vi "Main.vi"() -> ()   [LabVIEW 2020]
doc: "This template is for the Queued Message Handler design pattern.\n\nThe Event Handling Loop generates messages based on user interface actions.\n\nThe Message Handling Loop processes messages generated by the Event Handling Loop, or by other messages. The messages are string values, so new messages can be added easily to the Message Cases case structure in the Message Handling Loop. Each message cluster can also provide an optional value for Message Data, which is a variant that can be converted to whatever message-specific data is required."
uses:
  controls/UI Data.ctl
  controls/Lock-in config.ctl
  controls/Mono config.ctl
  <vilib>/event_ctls.llb/lveventtype.ctl
  Lock-in-amplifier/Libraries/Lock-in amplifier/Support/Filter config -- cluster.ctl
  Lock-in-amplifier/Libraries/Lock-in amplifier/Support/Input signal config -- typedef.ctl
  Lock-in-amplifier/Libraries/Lock-in amplifier/Support/Sense-Reserve config -- cluster.ctl
  controls/Wake HL data -- cluster.ctl
  <vilib>/Utility/sysdir.llb/System Directory Type.ctl
  support/Message Queue/Enqueue Message (Single).vi
  <vilib>/Utility/error.llb/Error Cluster From Error Code.vi
  <vilib>/ErrorRing/Error Ring.xnode
  support/Message Queue/Message Queue.lvlib
  support/User Event - Stop/User Event - Stop.lvlib
  Lock-in-amplifier/Libraries/Lock-in amplifier/Lock-in amplifier.lvlib
  Monochromator/Libraries/Monochromator/Monochromator.lvlib
panel:
  in  "Export":bool
  out "Current measurement":dbl caption="Medición" format="%0.6fmV"
  in  "Continous acquisition":bool
  in  "Simulate \nmono?":bool
  out "Last measurement":dbl caption="Medición" format="%#_gmV"
  in  "Position":dbl caption="Posición" format="%#_gnm"
  in  "Move":bool
  in  "Interval":dbl=10.0 caption="Intervalo" format="%#_gnm"
  out "Current position":dbl caption="Posición actual" format="%#_gnm"
  in  "Stop acquisition":bool
  out "XY Graph":cluster{"X":dbl, "Y":dbl}[](graph)
  in  "N samples":i32=1 caption="Muestras"
  in  "Average":bool
  in  "Final wavelength":dbl=800.0 caption="Fin" format="%#_gnm"
  in  "Initial wavelength":dbl=400.0 caption="Inicio" format="%#_gnm"
  in  "Speed":dbl=100.0 caption="Velocidad" format="%#_gnm/min"
  in  "Start acquiring":bool
  in  "Simulate \nlock-in?":bool
  out "Mono connected":bool
  out "Lock-in connected":bool
  in  "Settings":bool
  out "Status":string caption="Estado"
  in  "Exit":bool
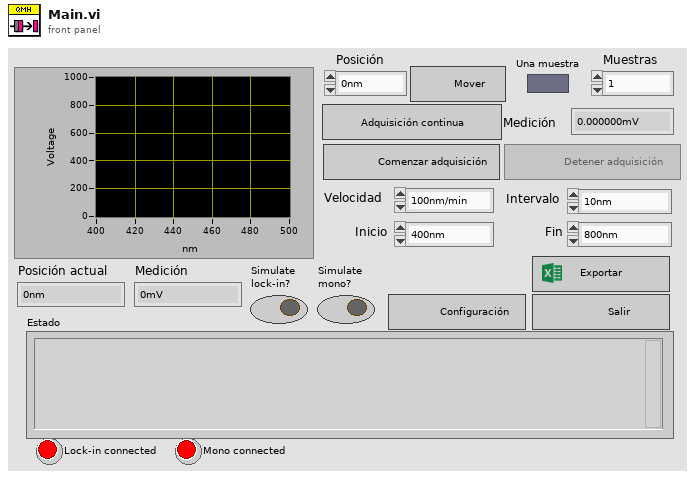
[diagram p1: front panel]
types:
  T1 = typedef "UI Data.ctl" = cluster{"Status":string, "Lockin Mod ID":i32, "Mono Mod ID":i32, "Lock-in config":T2, "Mono config":T3, "Lock-in connected?":bool, "Mono connected?":bool, "Data":cluster{"Position":dbl, "Value":dbl}[], "Manual move?":bool, "Current position":dbl, "Interval":dbl, "Operative?":bool}
  T2 = typedef "Lock-in config.ctl" = cluster{"VISA resource ":refnum<visa-resource-name>}
  T3 = typedef "Mono config.ctl" = cluster{"VISA resource ":refnum<visa-resource-name>, "nm/min":dbl}
  T4 = typedef "Lock-in amplifier.lvlib/Broadcast Events--cluster.ctl" = cluster{"Module Did Init":refnum<user-event>, "Status Updated":refnum<user-event>, "Error Reported":refnum<user-event>, "Module Did Stop":refnum<user-event>, "Update Module Execution Status":refnum<user-event>, "Helper Loop Status Updated":refnum<user-event>, "Data available":refnum<user-event>}
  T5 = typedef "Monochromator.lvlib/Broadcast Events--cluster.ctl" = cluster{"Module Did Init":refnum<user-event>, "Status Updated":refnum<user-event>, "Error Reported":refnum<user-event>, "Module Did Stop":refnum<user-event>, "Update Module Execution Status":refnum<user-event>, "Helper Loop Status Updated":refnum<user-event>, "Data read":refnum<user-event>, "GOTO ended":refnum<user-event>}
  T6 = cluster{"Stop Event":refnum<user-event>, "Wake HL":refnum<user-event>, "Stop HL":refnum<user-event>}
  T7 = typedef "Message Queue.lvlib/All Message Queues.ctl" = cluster{"UI":refnum<queue>}
  T8 = enum8{"Enabled", "Disabled", "Disabled and Grayed Out"}
  T9 = typedef "Wake HL data -- cluster.ctl" = cluster{"Mono Mod ID":i32, "Timeout":i32, "Wavelength":dbl}
  T10 = typedef "Lock-in amplifier.lvlib/Sense-Reserve config -- cluster.ctl" = cluster{"Dynamic Reserve ":i16, "Sensitivity":i16}
  T11 = typedef "Lock-in amplifier.lvlib/Input signal config -- typedef.ctl" = cluster{"Input Shield Grounding":u16, "Input Connection":u16, "Input Coupling":u16}
  T12 = typedef "Lock-in amplifier.lvlib/Filter config -- cluster.ctl" = cluster{"Time Constant":u16, "Enable Sync Filter?":bool, "Low Pass Filter Slope":u16}
  T13 = cluster{"baud rate":u32, "data bits":u16, "parity":enum16{"None", "Odd", "Even", "Mark", "Space"}, "stop bits":u16}
  T14 = typedef "System Directory Type.ctl" = i32
  T15 = typedef "lveventtype.ctl" = enum32{"Null", "Timeout", "Annotation Menu Selection", "Annotation Menu Selection?", "App Instance Close", "App Instance Close?", "Autoscale Range Change", "Bookmark Info Change", "Cell Edit", "Cell Edit?", "Cursor Grab", "Cursor Grab?", "Cursor Menu Selection", "Cursor Menu Selection?", "Cursor Move", "Cursor Release", "Data Change", "Direction Change", "Display State Change", "Drag Ended", "Drag Enter", "Drag Leave", "Drag Over", "Drag Source Update", "Drag Starting", "Drag Starting?", "Drop", "Exec State Change", "Key Down", "Key Down?", "Key Repeat", "Key Repeat?", "Key Up", "Listbox Double Click", "Menu Activation?", "Menu Selection (App)", "Menu Selection? (App)", "Menu Selection (User)", "Mouse Down", "Mouse Down?", "Mouse Enter", "Mouse Leave", "Mouse Move", "Mouse Up", "Mouse Wheel", "NI Security User Change (App)", "Pane Size", "Panel Close", "Panel Close?", "Panel Resize", "Plot Attribute Change", "Scale Range Change", "Shortcut Menu Activation?", "Shortcut Menu Selection (App)", "Shortcut Menu Selection? (App)", "Shortcut Menu Selection (User)", "Tree Double Click", "Tree Drag", "Tree Drag?", "Tree Drop", "Tree Drop?", "Tree Item Close", "Tree Item Close?", "Tree Item Open", "Tree Item Open?", "User Event", "Value Change"}
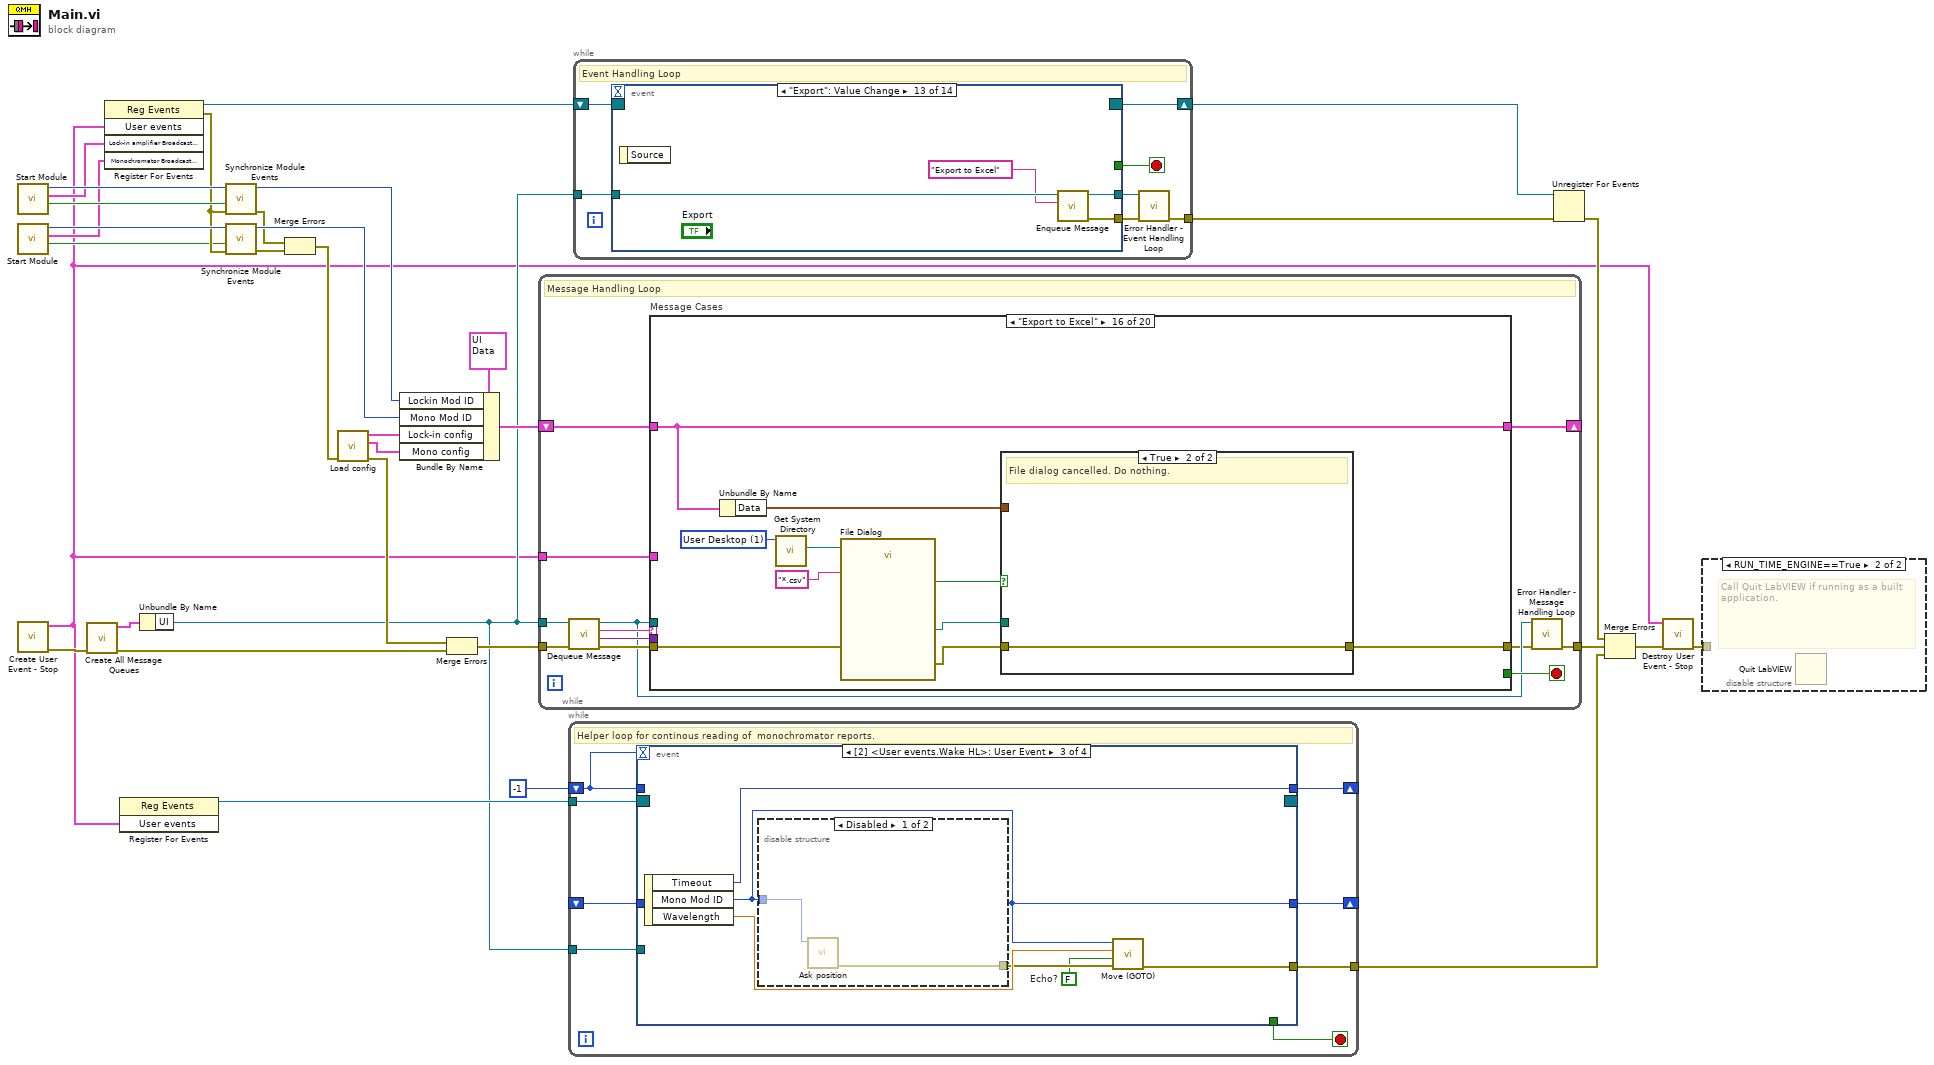
[diagram p0: block diagram]
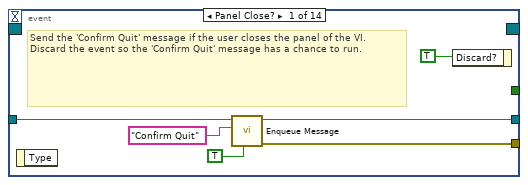
[diagram p2: hidden frame]
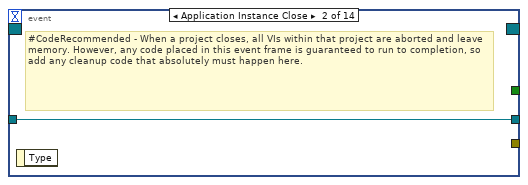
[diagram p3: hidden frame]
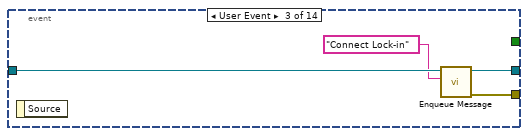
[diagram p4: hidden frame]
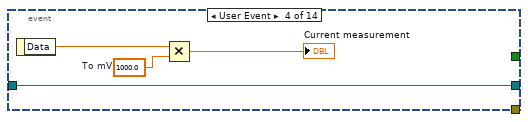
[diagram p5: hidden frame]
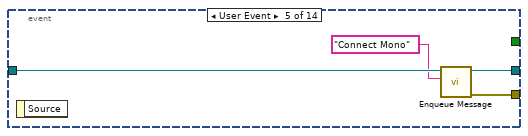
[diagram p6: hidden frame]
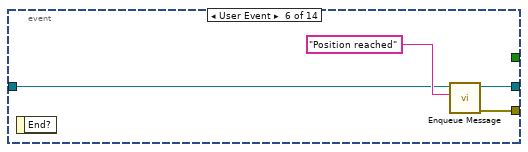
[diagram p7: hidden frame]
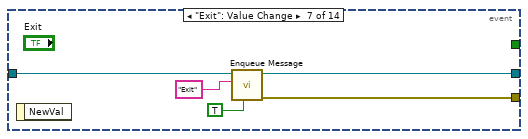
[diagram p8: hidden frame]
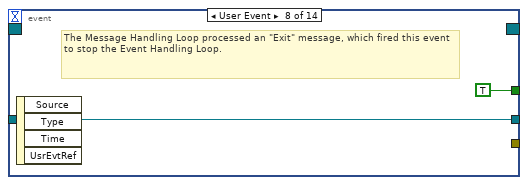
[diagram p9: hidden frame]
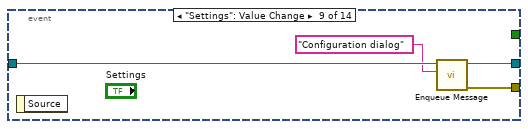
[diagram p10: hidden frame]
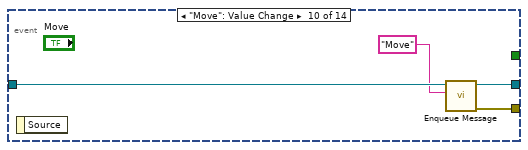
[diagram p11: hidden frame]
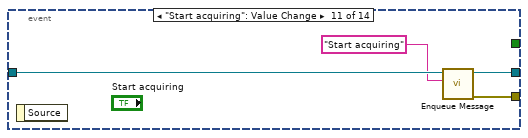
[diagram p12: hidden frame]
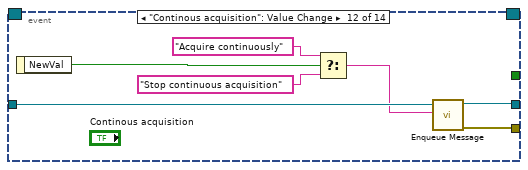
[diagram p13: hidden frame]
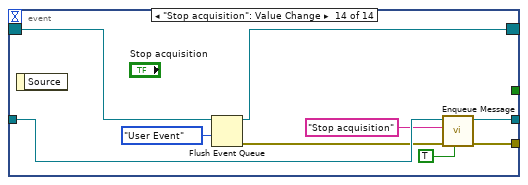
[diagram p14: hidden frame]
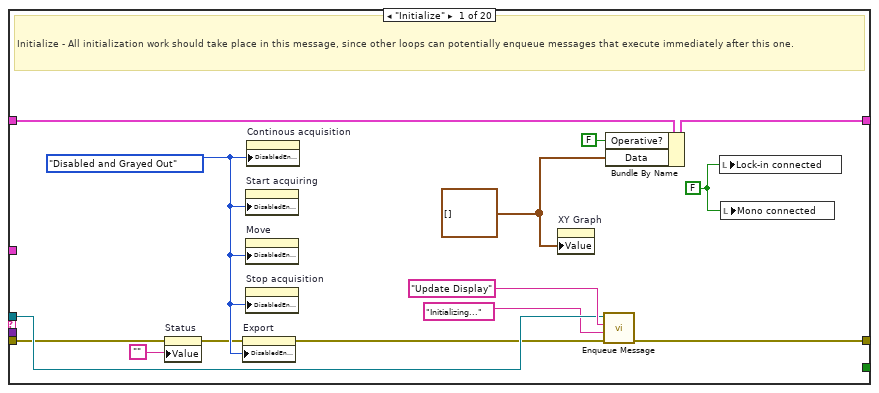
[diagram p15: hidden frame]
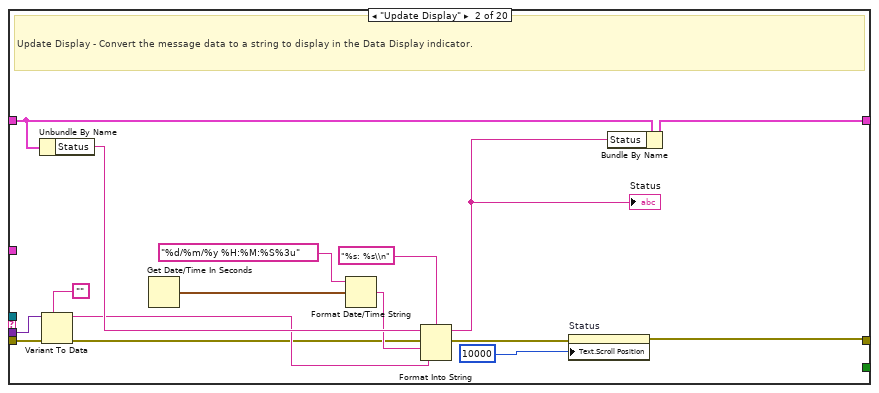
[diagram p16: hidden frame]
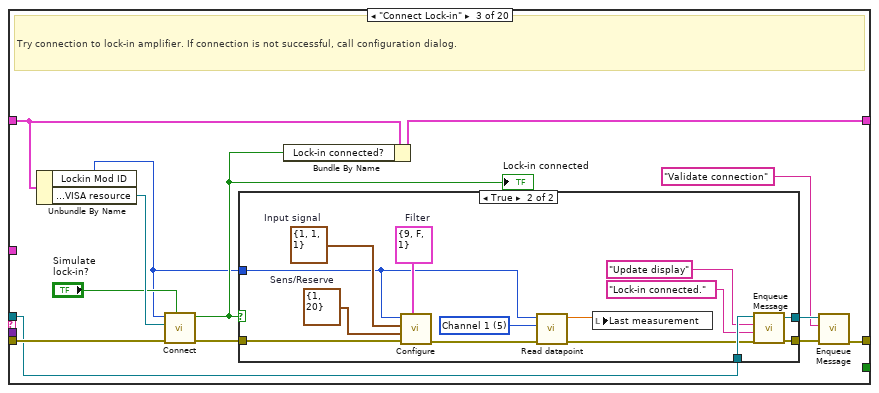
[diagram p17: hidden frame]
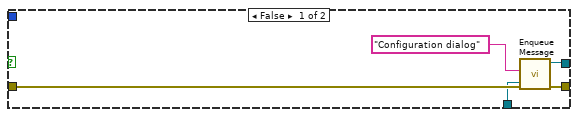
[diagram p18: hidden frame]
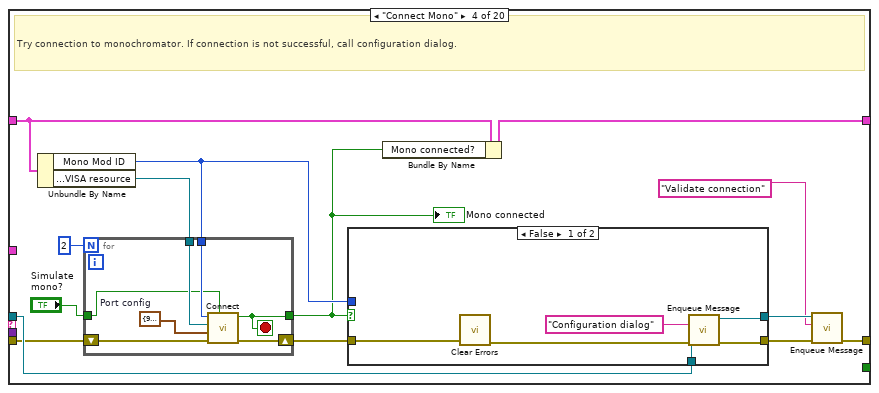
[diagram p19: hidden frame]
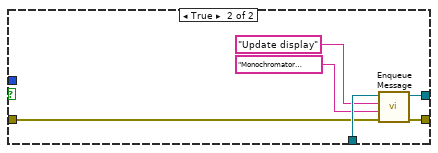
[diagram p20: hidden frame]
diagram:
  n1 = call "Start Module.vi"() -> ("Wait for Event Sync?"=w21:bool, "Lock-in amplifier Broadcast Events"=w20:T4, "Module ID"=w22:i32)  [unwired: 8 in, 1 out]
  n2 = call "Start Module.vi"() -> ("Wait for Event Sync?"=w16:bool, "Monochromator Broadcast Events"=w17:T5, "Module ID"=w19:i32)  [unwired: 8 in, 1 out]
  n3 = call "Create User Event - Stop.vi"() -> ("error out"=w30:errorcluster, "User events"=w1:T6)  [unwired: 10 in]
  n4 = call "Create All Message Queues.vi"("error in (no error)"=w30) -> ("error out"=w33:errorcluster, "Message Queues out"=w32:T7)  [unwired: 9 in]
  n5 = register-events(w1, w20, w17) -> (reference out=w24:refnum<event-registration>, error out=w18:errorcluster)  [unwired: 2 in]
  n6 = register-events(w1) -> (reference out=w4:refnum<event-registration>)  [unwired: 2 in, 1 out]
  n7 = Unbundle By Name(w32) -> ("UI"=w3:refnum<queue>)
  n8 = call "Synchronize Module Events.vi"("error in"=w18, "Wait for Event Sync?"=w21, "Module ID in"=w22) -> ("error out"=w11:errorcluster, "Module ID out"=w13:i32)  [unwired: 7 in]
  n9 = call "Synchronize Module Events.vi"("error in"=w18, "Wait for Event Sync?"=w16, "Module ID in"=w19) -> ("error out"=w10:errorcluster, "Module ID out"=w12:i32)  [unwired: 7 in]
  n10 = Merge Errors(w11, w10) -> (w9:errorcluster)
  n11 = call "Load config.vi"("error in (no error)"=w9) -> ("error out"=w8:errorcluster, "Mono config"=w6:T3, "Lock-in config"=w7:T2)  [unwired: 8 in]
  n12 = Bundle By Name(cluster=T1 {"Status"="", "Lockin Mod ID"=-1, "Mono Mod ID"=-1, "Lock-in config"={"VISA resource "=""}, "Mono config"={"VISA resource "="", "nm/min"=0.0}, "Lock-in connected?"=FALSE, "Mono connected?"=FALSE, "Data"=[], "Manual move?"=FALSE, "Current position"=0.0, "Interval"=0.0, "Operative?"=FALSE} ("Data Cluster"), "Lockin Mod ID"=w13, "Mono Mod ID"=w12, "Lock-in config"=w7, "Mono config"=w6) -> (w14:T1)
  n13 = Merge Errors(w8, w33) -> (w23:errorcluster)
  n14 = while {
    tunnel: w3 -> [w37]
    shift-right: [w44] -> _
    shift-left: w14 -> [w45]
    tunnel: w1 -> [w42]
    tunnel: w23 -> [w41]
    tunnel: [w35] -> w31
    stop <- w43 stop-if-true
    # "Message Handling Loop"
    n15 = call "Dequeue Message.vi"("error in (no error)"=w41, "Message Queue"=w37) -> ("error out"=w40:errorcluster, "Message Data"=w38:variant, "Message"=w39:string, "dup Message Queue"=w36:refnum<queue>)  [unwired: 6 in]
    n16 = case "Message Cases" shown="\"Export to Excel\"" w39 {
      selector: w39 -> [_ _ _ _ _ _ _ _ _ _ _ _ _ _ _ _ _ _ _ w392]
      tunnel: w36 -> [w57 _ w85 w121 w147 w175 w209 w233 _ _ _ w270 w285 w296 w323 _ _ w372 w391 _]
      tunnel: w40 -> [w51 w75 w88 w120 w149 w180 w222 w230 w248 w253 w257 w267 w294 w305 w333 w357 w369 w376 w387 _]
      tunnel: [w59 w65 w78 w111 w148 w174 w210 w234 w247 w252 w262 w271 w291 w304 w332 w351 w363 w374 w388 w393] -> w34
      tunnel: w45 -> [w55 w63 w84 w116 w143 w182 w214 w229 w246 w251 w260 w264 w282 w300 w336 w350 w368 w375 w380 w394]
      tunnel: [w53 w62 w83 w115 w142 w181 w212 w229 w246 w251 w258 w263 w282 w302 w334 w350 w368 w375 w380 w394] -> w44
      tunnel: [_ _ _ _ _ _ _ _ _ _ _ _ _ _ _ _ _ _ TRUE _] -> w43
      tunnel: w38 -> [_ w74 _ _ _ _ _ _ _ _ _ _ _ _ w329 _ w367 _ w384 _]
      tunnel: w42 -> [_ _ _ _ _ _ w220 _ _ _ _ _ w295 w301 w330 _ _ _ w377 _]
      frame "Initialize" {
        w52 = FALSE ("Lock-in connected")
        w48 = T8."Disabled and Grayed Out" ("Disabled")
        w54 = cluster{"Position":dbl, "Value":dbl}[] [] ("Data")
        # "Initialize - All initialization work should take place in this message, since other loops can potentially enqueue messages that execute immediately after this one."
        n17 = property on="Status" class="Str"(error in=w51, "Value"="") -> (error out=w47:errorcluster)  [unwired: 1 in, 1 out]
        n18 = property on="Export" class="Bool"(error in=w47, "DisabledEnum"=w48) -> (error out=w46:errorcluster)  [unwired: 1 in, 1 out]
        n19 = property on="Start acquiring" class="Bool"("DisabledEnum"=w48) -> ()  [unwired: 2 in, 2 out]
        n20 = property on="Move" class="Bool"("DisabledEnum"=w48) -> ()  [unwired: 2 in, 2 out]
        n21 = property on="Stop acquisition" class="Bool"("DisabledEnum"=w48) -> ()  [unwired: 2 in, 2 out]
        n22 = property on="Continous acquisition" class="Bool (strict)"("DisabledEnum"=w48) -> ()  [unwired: 2 in, 2 out]
        n23 = property on="XY Graph" class="XYGraph (strict)"("Value"=w54) -> ()  [unwired: 2 in, 2 out]
        n24 = call-poly "Enqueue Message.vi"("error in (no error)"=w46, "Message Data"="Initializing..." ("Initial Message"), "Message"="Update Display", "Message Queue"=w57) -> ("error out"=w59:errorcluster)  [unwired: 6 in, 1 out]
        n25 = Bundle By Name(cluster=w55, "Operative?"=FALSE, "Data"=w54) -> (w53:T1)
        n26 = local write "Lock-in connected"(w52) -> ()
        n27 = local write "Mono connected"(w52) -> ()
      }
      frame "Update Display" {
        # "Update Display - Convert the message data to a string to display in the Data Display indicator."
        n28 = Unbundle By Name(w63) -> ("Status"=w72:string)
        n29 = Variant To Data(error in=w75, type="", Variant=w74) -> (data=w68:string, error out=w67:errorcluster)
        n30 = Get Date/Time In Seconds() -> (seconds since 1Jan1904=w70:timestamp)
        n31 = Format Date/Time String(time format string (%c)="%d/%m/%y %H:%M:%S%3u", seconds (now)=w70) -> (date/time string=w69:string)  [unwired: 1 in]
        n32 = Format Into String(format string="%s: %s\\n", initial string=w72, error in=w67, w69, w68) -> (resulting string=w61:string, error out=w66:errorcluster)
        "Status" <- w61
        n33 = property on="Status" class="Str"(error in=w66, "Text.Scroll Position"=u32 10000) -> (error out=w65:errorcluster)  [unwired: 1 in, 1 out]
        n34 = Bundle By Name(cluster=w63, "Status"=w61) -> (w62:T1)
      }
      frame "Connect Lock-in" {
        # "Try connection to lock-in amplifier. If connection is not successful, call configuration dialog."
        n35 = Unbundle By Name(w84) -> ("Lockin Mod ID"=w80:i32, "Lock-in config.VISA resource"=w87:refnum<visa-resource-name>)
        n36 = call "Connect.vi"("Simulate?"="Simulate \nlock-in?", "error in"=w88, "VISA resource name"=w87, "Module ID"=w80) -> ("error out"=w86:errorcluster, "Connection successful?"=w82:bool)  [unwired: 5 in, 1 out]
        "Lock-in connected" <- w82
        n37 = case shown="True" w82 {
          tunnel: w86 -> [w92 w103]
          tunnel: [w93 w104] -> w79
          tunnel: w85 -> [w91 w107]
          tunnel: w80 -> [_ w97]
          tunnel: [w89 w94] -> w77
          frame False {
            n38 = call-poly "Enqueue Message.vi"("error in (no error)"=w92, "Message"="Configuration dialog", "Message Queue"=w91) -> ("error out"=w93:errorcluster, "dup Message Queue"=w89:refnum<queue>)  [unwired: 7 in]
          }
          frame True {
            w96 = u16 5 items=["X"=1, "Y"=2, "R"=3, "Theta"=4, "Channel 1"=5, "Channel 2"=6, "Aux In 1"=7, "Aux In 2"=8, "Aux In 3"=9, "Aux In 4"=10] ("Parameter")
            w100 = T10 {"Dynamic Reserve "=1, "Sensitivity"=20}  # Sens/Reserve
            w101 = T11 {"Input Shield Grounding"=1, "Input Connection"=1, "Input Coupling"=1}  # Input signal
            w102 = T12 {"Time Constant"=9, "Enable Sync Filter?"=FALSE, "Low Pass Filter Slope"=1}  # Filter
            n39 = call "Configure.vi"("Filter"=w102, "error in"=w103, "Sens/Reserve"=w100, "Input signal"=w101, "Module ID"=w97) -> ("error out"=w99:errorcluster)  [unwired: 6 in]
            n40 = call "Read datapoint.vi"("error in"=w99, "Parameter"=w96, "Module ID"=w97) -> ("error out"=w98:errorcluster, "Data"=w95:dbl)  [unwired: 6 in, 1 out]
            n41 = local write "Last measurement"(w95) -> ()
            n42 = call-poly "Enqueue Message.vi"("error in (no error)"=w98, "Message Data"="Lock-in connected." ("Message"), "Message"="Update display", "Message Queue"=w107) -> ("error out"=w104:errorcluster, "dup Message Queue"=w94:refnum<queue>)  [unwired: 6 in]
          }
        }
        n43 = Bundle By Name(cluster=w84, "Lock-in connected?"=w82) -> (w83:T1)
        n44 = call-poly "Enqueue Message.vi"("error in (no error)"=w79, "Message"="Validate connection", "Message Queue"=w77) -> ("error out"=w78:errorcluster)  [unwired: 7 in, 1 out]
      }
      frame "Connect Mono" {
        # "Try connection to monochromator. If connection is not successful, call configuration dialog."
        n45 = Unbundle By Name(w116) -> ("Mono Mod ID"=w117:i32, "Mono config.VISA resource"=w119:refnum<visa-resource-name>)
        n46 = for {
          N: 2 -> [_]
          tunnel: w119 -> [w127]
          tunnel: w117 -> [w125]
          shift-right: [w126] -> w118
          shift-left: w120 -> [w128]
          tunnel: "Simulate \nmono?" -> [w123]
          tunnel: [w122] -> w108
          stop <- w122 stop-if-true
          w124 = T13 {"baud rate"=9600, "data bits"=8, "parity"=enum."None", "stop bits"=10}  # Port config
          n47 = call "Connect.vi"("Simulate?"=w123, "error in"=w128, "Port config"=w124, "VISA resource name"=w127, "Module ID"=w125) -> ("error out"=w126:errorcluster, "Connected?"=w122:bool)  [unwired: 4 in, 1 out]
        }
        "Mono connected" <- w108
        n48 = case shown="False" w108 {
          tunnel: w118 -> [w131 w135]
          tunnel: [w134 w140] -> w112
          tunnel: w121 -> [w133 w139]
          tunnel: w117 -> [_ _]
          tunnel: [w129 w136] -> w110
          frame False {
            n49 = call <vilib>:"Clear Errors.vi"("error in (no error)"=w131) -> ("error out"=w130:errorcluster)  [unwired: 5 in, 1 out]
            n50 = call-poly "Enqueue Message.vi"("error in (no error)"=w130, "Message"="Configuration dialog", "Message Queue"=w133) -> ("error out"=w134:errorcluster, "dup Message Queue"=w129:refnum<queue>)  [unwired: 7 in]
          }
          frame True {
            n51 = call-poly "Enqueue Message.vi"("error in (no error)"=w135, "Message Data"="Monochromator connected." ("Message"), "Message"="Update display", "Message Queue"=w139) -> ("error out"=w140:errorcluster, "dup Message Queue"=w136:refnum<queue>)  [unwired: 6 in]
          }
        }
        n52 = Bundle By Name(cluster=w116, "Mono connected?"=w108) -> (w115:T1)
        n53 = call-poly "Enqueue Message.vi"("error in (no error)"=w112, "Message"="Validate connection", "Message Queue"=w110) -> ("error out"=w111:errorcluster)  [unwired: 7 in, 1 out]
      }
      frame "Validate connection" {
        # "If both devices establish correct communication, enable operating controls."
        n54 = Unbundle By Name(w143) -> ("Operative?"=w145:bool, "Mono Mod ID"=w146:i32)
        n55 = local read "Lock-in connected"() -> (w150:bool)
        n56 = local read "Mono connected"() -> (w151:bool)
        n57 = Not(x=w145) -> (.not. x?=w144:bool)
        n58 = Compound Arithmetic op=AND(w144, w151, w150) -> (w152:bool)
        n59 = case shown="True" w152 {
          tunnel: w149 -> [w153 w157]
          tunnel: [w153 w166] -> w148
          tunnel: w147 -> [_ w165]
          tunnel: w146 -> [_ w155]
          tunnel: [_ TRUE] -> w141
          frame False {
          }
          frame True {
            w167 = T8."Enabled" ("Disabled")
            n60 = call "Move (GOTO).vi"("error in"=w157, "Echo?"=TRUE, "Position"=0.0, "Module ID"=w155) -> ("error out"=w161:errorcluster)  [unwired: 5 in, 2 out]
            n61 = for {
              N: 2 -> [_]
              tunnel: w155 -> [w169]
              tunnel: [w168] -> w162
              shift-right: [w170] -> w156
              shift-left: w161 -> [w171]
              n62 = call "Ask position.vi"("error in"=w171, "Module ID"=w169) -> ("error out"=w170:errorcluster, "Current position"=w168:dbl)  [unwired: 7 in, 1 out]
            }
            n63 = local write "Current position"(w162) -> ()
            n64 = property on="Start acquiring" class="Bool"("DisabledEnum"=w167) -> ()  [unwired: 2 in, 2 out]
            n65 = property on="Move" class="Bool"("DisabledEnum"=w167) -> ()  [unwired: 2 in, 2 out]
            n66 = property on="Continous acquisition" class="Bool (strict)"("DisabledEnum"=w167) -> ()  [unwired: 2 in, 2 out]
            n67 = call-poly "Enqueue Message.vi"("error in (no error)"=w156, "Message Data"="Homing..." ("Message"), "Message"="Update display", "Message Queue"=w165) -> ("error out"=w166:errorcluster)  [unwired: 6 in, 1 out]
          }
        }
        n68 = Bundle By Name(cluster=w143, "Operative?"=w141) -> (w142:T1)
      }
      frame "Configuration dialog" {
        n69 = Unbundle By Name(w182) -> ("Lock-in config"=w184:T2, "Mono config"=w183:T3, "Mono Mod ID"=w176:i32, "Lockin Mod ID"=w177:i32)
        n70 = call "Config dialog.vi"("error in (no error)"=w180, "Mono config"=w183, "Lock-in config"=w184) -> ("error out"=w179:errorcluster, "Cancelled?"=w178:bool, "Mono config out"=w172:T3, "Lock-in config out"=w173:T2)  [unwired: 5 in]
        n71 = case shown="True" w178 {
          tunnel: w179 -> [w198 w199]
          tunnel: w177 -> [w197 _]
          tunnel: w176 -> [w195 _]
          tunnel: w175 -> [w193 _]
          tunnel: [w189 w199] -> w174
          tunnel: w173 -> [w186 _]
          tunnel: w172 -> [w185 _]
          frame False {
            # "Dialog not cancelled. Reconfigure."
            n72 = call "Disconnect.vi"("error in"=w198, "Module ID"=w197) -> ("error out"=w196:errorcluster)  [unwired: 9 in]
            n73 = call "Disconnect.vi"("error in"=w196, "Module ID"=w195) -> ("error out"=w188:errorcluster)  [unwired: 9 in]
            n74 = call "Save config.vi"("error in (no error)"=w188, "Mono config"=w185, "Lock-in config"=w186) -> ("error out"=w187:errorcluster)  [unwired: 8 in]
            n75 = call-poly "Enqueue Message.vi"("error in (no error)"=w187, "Message"="Connect Lock-in", "Message Queue"=w193) -> ("error out"=w192:errorcluster, "dup Message Queue"=w191:refnum<queue>)  [unwired: 7 in]
            n76 = call-poly "Enqueue Message.vi"("error in (no error)"=w192, "Message"="Connect Mono", "Message Queue"=w191) -> ("error out"=w189:errorcluster)  [unwired: 7 in, 1 out]
          }
          frame True {
            # "Dialog cancelled. Do nothing."
          }
        }
        n77 = Bundle By Name(cluster=w182, "Lock-in config"=w173, "Mono config"=w172) -> (w181:T1)
      }
      frame "Start acquiring" {
        w200 = T8."Disabled and Grayed Out" ("Disabled")
        w213 = cluster{"Position":dbl, "Value":dbl}[] [] ("Data")
        n78 = Unbundle By Name(w214) -> ("Mono Mod ID"=w206:i32)
        n79 = Unbundle By Name(w220) -> ("Wake HL"=w219:refnum<user-event>)
        n80 = call "Configure movement.vi"("Final wavelength"="Final wavelength", "error in (no error)"=w222, "Initial wavelength"="Initial wavelength", "Mono Mod ID"=w206, "Speed"="Speed") -> ("error out"=w215:errorcluster)  [unwired: 6 in]
        n81 = Bundle By Name(cluster=T9 {"Mono Mod ID"=0, "Timeout"=0, "Wavelength"=0.0} ("Wake HL"), "Wavelength"="Initial wavelength", "Mono Mod ID"=w206, "Timeout"=300) -> (w217:T9)
        n82 = Bundle By Name(cluster=w214, "Current position"="Initial wavelength", "Interval"="Interval", "Manual move?"=FALSE, "Data"=w213) -> (w212:T1)
        n83 = property on="XY Graph" class="XYGraph (strict)"("Value"=w213, "XScale.Minimum"="Initial wavelength", "XScale.Maximum"="Final wavelength") -> ()  [unwired: 2 in, 2 out]
        n84 = Generate User Event(user event=w219, event data cluster=w217, error in=w215) -> (error out=w211:errorcluster)  [unwired: 1 in, 1 out]
        n85 = call-poly "Enqueue Message.vi"("error in (no error)"=w211, "Message Data"="Acquisition started." ("Message"), "Message"="Update Display", "Message Queue"=w209) -> ("error out"=w210:errorcluster)  [unwired: 6 in, 1 out]
        n86 = property on="Move" class="Bool"("DisabledEnum"=w200) -> ()  [unwired: 2 in, 2 out]
        n87 = property on="Start acquiring" class="Bool"("DisabledEnum"=w200) -> ()  [unwired: 2 in, 2 out]
        n88 = property on="Continous acquisition" class="Bool (strict)"("DisabledEnum"=w200) -> ()  [unwired: 2 in, 2 out]
        n89 = property on="Stop acquisition" class="Bool"("DisabledEnum"=T8."Enabled" ("Disabled")) -> ()  [unwired: 2 in, 2 out]
        n90 = property on="Export" class="Bool"("DisabledEnum"=w200) -> ()  [unwired: 2 in, 2 out]
        "Current position" <- "Initial wavelength"
      }
      frame "Acquisition complete" {
        n91 = Unbundle By Name(w229) -> ("Mono Mod ID"=w228:i32)
        n92 = call "Move (GOTO).vi"("error in"=w230, "Echo?"=FALSE, "Position"=0.0, "Module ID"=w228) -> ("error out"=w225:errorcluster, "Done?"=w224:bool)  [unwired: 5 in, 1 out]
        n93 = property on="Stop acquisition" class="Bool"("DisabledEnum"=T8."Disabled and Grayed Out" ("Disabled")) -> ()  [unwired: 2 in, 2 out]
        n94 = case shown="True" w224 {
          tunnel: w225 -> [w237 w239]
          tunnel: [w237 w239] -> w223
          frame False {
          }
          frame True {
            w238 = T8."Enabled" ("Disabled")
            n95 = property on="Start acquiring" class="Bool"("DisabledEnum"=w238) -> ()  [unwired: 2 in, 2 out]
            n96 = property on="Move" class="Bool"("DisabledEnum"=w238) -> ()  [unwired: 2 in, 2 out]
            n97 = property on="Continous acquisition" class="Bool (strict)"("DisabledEnum"=w238) -> ()  [unwired: 2 in, 2 out]
            n98 = property on="Export" class="Bool"("DisabledEnum"=w238) -> ()  [unwired: 2 in, 2 out]
          }
        }
        n99 = One Button Dialog(message="Se ha completado la adquisición.") -> ()  [unwired: 1 in, 1 out]
        n100 = call-poly "Enqueue Message.vi"("error in (no error)"=w223, "Message Data"="Acquition completed. Homing..." ("Message"), "Message"="Update display", "Message Queue"=w233) -> ("error out"=w234:errorcluster)  [unwired: 6 in, 1 out]
      }
      frame "Acquire continuously" {
        w242 = u16 5 items=["X"=1, "Y"=2, "R"=3, "Theta"=4, "Channel 1"=5, "Channel 2"=6, "Aux In 1"=7, "Aux In 2"=8, "Aux In 3"=9, "Aux In 4"=10] ("Parameter")
        n101 = Unbundle By Name(w246) -> ("Lockin Mod ID"=w245:i32)
        n102 = local read "Average"() -> (w244:bool)
        n103 = local read "N samples"() -> (w243:i32)
        n104 = call "Start continuous acquisition.vi"("N-samples"=w243, "Timeout"=100, "Average?"=w244, "error in"=w248, "Parameter"=w242, "Module ID"=w245) -> ("error out"=w247:errorcluster)  [unwired: 5 in]
        n105 = property on="Start acquiring" class="Bool"("DisabledEnum"=T8."Disabled and Grayed Out" ("Disabled")) -> ()  [unwired: 2 in, 2 out]
      }
      frame "Stop continuous acquisition" {
        n106 = Unbundle By Name(w251) -> ("Lockin Mod ID"=w250:i32)
        n107 = call "Stop continuous acquisition.vi"("error in"=w253, "Module ID"=w250) -> ("error out"=w252:errorcluster)  [unwired: 9 in]
        n108 = property on="Start acquiring" class="Bool"("DisabledEnum"=T8."Enabled" ("Disabled")) -> ()  [unwired: 2 in, 2 out]
      }
      frame "Move" {
        w261 = T8."Disabled and Grayed Out" ("Disabled")
        n109 = Unbundle By Name(w260) -> ("Mono Mod ID"=w256:i32)
        n110 = call "Move (GOTO).vi"("error in"=w257, "Echo?"=TRUE, "Position"="Position", "Module ID"=w256) -> ("error out"=w262:errorcluster)  [unwired: 5 in, 2 out]
        n111 = property on="Continous acquisition" class="Bool (strict)"("DisabledEnum"=w261) -> ()  [unwired: 2 in, 2 out]
        n112 = property on="Start acquiring" class="Bool"("DisabledEnum"=w261) -> ()  [unwired: 2 in, 2 out]
        n113 = property on="Stop acquisition" class="Bool"("DisabledEnum"=w261) -> ()  [unwired: 2 in, 2 out]
        n114 = Bundle By Name(cluster=w260, "Manual move?"=TRUE) -> (w258:T1)
      }
      frame "Position reached" {
        n115 = Unbundle By Name(w264) -> ("Manual move?"=w272:bool, "Mono Mod ID"=w265:i32)
        n116 = case shown="True" w272 {
          tunnel: w267 -> [w274 w280]
          tunnel: [w274 w279] -> w266
          tunnel: w265 -> [_ w278]
          tunnel: w264 -> [w273 w277]
          tunnel: [w273 w276] -> w263
          frame False {
          }
          frame True {
            w281 = T8."Enabled" ("Disabled")
            n117 = property on="Start acquiring" class="Bool"("DisabledEnum"=w281) -> ()  [unwired: 2 in, 2 out]
            n118 = property on="Continous acquisition" class="Bool (strict)"("DisabledEnum"=w281) -> ()  [unwired: 2 in, 2 out]
            n119 = call "Ask position.vi"("error in"=w280, "Module ID"=w278) -> ("error out"=w279:errorcluster, "Current position"=w275:dbl)  [unwired: 7 in, 1 out]
            n120 = Bundle By Name(cluster=w277, "Current position"=w275) -> (w276:T1)
            n121 = local write "Current position"(w275) -> ()
          }
        }
        n122 = call-poly "Enqueue Message.vi"("error in (no error)"=w266, "Message Data"="Position reached" ("Message"), "Message"="Update display", "Message Queue"=w270) -> ("error out"=w271:errorcluster)  [unwired: 6 in, 1 out]
      }
      frame "Stop acquisition" {
        w288 = T8."Enabled" ("Disabled")
        n123 = Unbundle By Name(w295) -> ("Stop HL"=w293:refnum<user-event>)
        n124 = Generate User Event(user event=w293, event data cluster=FALSE ("event data"), error in=w294) -> (error out=w283:errorcluster)  [unwired: 1 in, 1 out]
        n125 = property on="Stop acquisition" class="Bool"("DisabledEnum"=T8."Disabled and Grayed Out" ("Disabled")) -> ()  [unwired: 2 in, 2 out]
        n126 = Flush Queue(queue=w285, error in (no error)=w283) -> (queue out=w284:refnum<queue>, error out=w286:errorcluster)  [unwired: 1 out]
        n127 = property on="Start acquiring" class="Bool"("DisabledEnum"=w288) -> ()  [unwired: 2 in, 2 out]
        n128 = property on="Move" class="Bool"("DisabledEnum"=w288) -> ()  [unwired: 2 in, 2 out]
        n129 = property on="Continous acquisition" class="Bool (strict)"("DisabledEnum"=w288) -> ()  [unwired: 2 in, 2 out]
        n130 = call-poly "Enqueue Message.vi"("error in (no error)"=w286, "Message Data"="Acquisition stopped." ("Message"), "Message"="Update Display", "Message Queue"=w284) -> ("error out"=w291:errorcluster)  [unwired: 6 in, 1 out]
      }
      frame "Acquire data" {
        n131 = local read "Final wavelength"() -> (w298:dbl)
        n132 = Unbundle By Name(w300) -> ("Current position"=w299:dbl)
        n133 = Less Or Equal?(x=w299, y=w298) -> (x <= y?=w297:bool)
        n134 = case shown="True" w297 {
          tunnel: "Average" -> [_ w322]
          tunnel: w300 -> [w311 w321]
          tunnel: w305 -> [w310 w320]
          tunnel: [w309 w316] -> w304
          tunnel: "N samples" -> [_ w319]
          tunnel: [w311 w318] -> w302
          tunnel: w301 -> [_ _]
          tunnel: w296 -> [w308 w315]
          frame False {
            n135 = call-poly "Enqueue Message.vi"("error in (no error)"=w310, "Message"="Acquisition complete", "Message Queue"=w308) -> ("error out"=w309:errorcluster)  [unwired: 7 in, 1 out]
          }
          frame True {
            n136 = call "Acquire data -- subVI.vi"("N samples"=w319, "error in (no error)"=w320, "Average"=w322, "Data Cluster"=w321) -> ("error out"=w313:errorcluster, "event data"=w312:T9, "Measurement"=→"Last measurement":dbl, "Data Cluster"=w318:T1)  [unwired: 4 in]
            n137 = call-poly "Enqueue Message.vi"("error in (no error)"=w313, "Message Data"=w312, "Message"="Update results", "Message Queue"=w315) -> ("error out"=w316:errorcluster)  [unwired: 6 in, 1 out]
          }
        }
      }
      frame "Update results" {
        n138 = Unbundle By Name(w336) -> ("Data"=→"XY Graph":cluster{"Position":dbl, "Value":dbl}[], "Interval"=w337:dbl, "Current position"=w325:dbl)  [unwired: 1 out]
        n139 = local read "Final wavelength"() -> (w326:dbl)
        n140 = Variant To Data(error in=w333, type=T9 {"Mono Mod ID"=0, "Timeout"=0, "Wavelength"=0.0} ("event data"), Variant=w329) -> (data=w327:T9, error out=w331:errorcluster)
        n141 = Less?(x=w325, y=w326) -> (x < y?=w324:bool)
        n142 = local write "Current position"(w325) -> ()
        n143 = Add(x=w337, y=w325) -> (x+y=w335:dbl)
        n144 = case shown="False" w324 {
          tunnel: [w340 w347] -> w332
          tunnel: w331 -> [w341 w346]
          tunnel: w330 -> [_ w345]
          tunnel: w327 -> [_ w343]
          tunnel: w323 -> [w339 _]
          frame False {
            n145 = call-poly "Enqueue Message.vi"("error in (no error)"=w341, "Message"="Acquisition complete", "Message Queue"=w339) -> ("error out"=w340:errorcluster)  [unwired: 7 in, 1 out]
          }
          frame True {
            n146 = Unbundle By Name(w345) -> ("Wake HL"=w344:refnum<user-event>)
            n147 = Generate User Event(user event=w344, event data cluster=w343, error in=w346) -> (error out=w347:errorcluster)  [unwired: 1 in, 1 out]
          }
        }
        n148 = Bundle By Name(cluster=w336, "Current position"=w335) -> (w334:T1)
      }
      frame "Export to Excel" {
        w356 = T14 1 items=["User Home"=0, "User Desktop"=1, "User Documents"=2, "User Application Data"=3, "User Preferences"=4, "User Temporary"=5, "Public Documents"=6, "Public Application Data"=7, "Public Preferences"=8, "Public Cache"=13, "System Core Libraries"=9, "System Installed Libraries"=10, "Application Files"=11, "Boot Volume Root"=12] ("system directory type")
        n149 = Unbundle By Name(w350) -> ("Data"=w349:cluster{"Position":dbl, "Value":dbl}[])
        n150 = call <vilib>:"Get System Directory.vi"("system directory type"=w356) -> ("system directory"=w355:path)  [unwired: 10 in]
        n151 = call "File Dialog"("start path"=w355, "error in"=w357, "pattern (all files)"="*.csv") -> ("selected path"=w348:path, "cancelled"=w353:bool, "error out"=w352:errorcluster)  [unwired: 9 in, 1 out]
        n152 = case shown="True" w353 {
          tunnel: w352 -> [w359 w362]
          tunnel: [w358 w362] -> w351
          tunnel: w349 -> [w361 _]
          tunnel: w348 -> [w360 _]
          frame False {
            # "File dialog not cancelled. Save to file."
            n153 = call "Format and write to Excel.vi"("error in (no error)"=w359, "Data"=w361, "selected path"=w360) -> ("error out"=w358:errorcluster)  [unwired: 8 in]
          }
          frame True {
            # "File dialog cancelled. Do nothing."
          }
        }
      }
      frame "Error" {
        # "Error - Display an error dialog. This message is sent by the \"Error Handler\" VIs at the end of other loops in this application."
        n154 = Variant To Data(error in=w369, type=errorcluster {"status"=FALSE, "code"=0, "source"=""} ("error constant"), Variant=w367) -> (data=w365:errorcluster, error out=w364:errorcluster)
        n155 = call <vilib>:"Simple Error Handler.vi"("error in (no error)"=w365) -> ()  [unwired: 4 in, 5 out]
        n156 = Merge Errors(w364) -> (w363:errorcluster)
      }
      frame "Confirm Quit" {
        # "#CodeNeeded - If you want to provide an \"Are you sure\" dialog (or some other notification) before the application exits, place that code here. This message is typically sent from a Panel Close? event."
        # "Confirm Quit - Message that can confirm whether or not the user wants to exit the application."
        n157 = call-poly "Enqueue Message.vi"("Priority Message? (F)"=TRUE, "error in (no error)"=w376, "Message"="Exit", "Message Queue"=w372) -> ("error out"=w373:errorcluster)  [unwired: 6 in, 1 out]
        n158 = Merge Errors(w373) -> (w374:errorcluster)
      }
      frame "Exit" {
        # "Exit - Exit the application."
        n159 = Variant To Data(type=errorcluster {"status"=FALSE, "code"=0, "source"=""} ("error constant"), Variant=w384) -> (data=w385:errorcluster)  [unwired: 1 in, 1 out]
        n160 = Unbundle By Name(w380) -> ("Mono Mod ID"=w378:i32, "Lockin Mod ID"=w379:i32)
        n161 = call <vilib>:"Simple Error Handler.vi"("error in (no error)"=w385) -> ()  [unwired: 4 in, 5 out]
        n162 = call "Fire User Event - Stop.vi"("User events"=w377) -> ("error out"=w383:errorcluster)  [unwired: 10 in]
        n163 = call "Stop Module.vi"("error in"=w383, "Module ID"=w379) -> ("error out"=w382:errorcluster)  [unwired: 9 in]
        n164 = Release Queue(queue=w391, error in (no error)=w387) -> (error out=w389:errorcluster)  [unwired: 1 in, 2 out]
        n165 = call "Stop Module.vi"("error in"=w382, "Module ID"=w378) -> ("error out"=w381:errorcluster)  [unwired: 9 in]
        n166 = Merge Errors(w381, w389) -> (w388:errorcluster)
      }
      frame Default {
        # "'Default' case only runs if there is a message that isn't defined in any of the other cases.  Output a programming error."
        n167 = xnode "Error Ring"("parameter 0"=w392) -> ("error out"=w393:errorcluster)
      }
    }
    n168 = call "Error Handler - Message Handling Loop.vi"("error in (no error)"=w34, "Message Queue"=w36) -> ("dup error in"=w35:errorcluster)  [unwired: 8 in, 1 out]
  }
  n169 = while {
    shift-right: [w406] -> _
    shift-left: -1 -> [w407]
    tunnel: w4 -> [w409]
    tunnel: w3 -> [w403]
    shift-right: [w405] -> _
    shift-left: _ -> [w404]
    tunnel: [w402] -> w2
    stop <- w408 stop-if-true
    # "Helper loop for continous reading of  monochromator reports."
    n170 = event shown="[2] <User events.Wake HL>: User Event" {
      selector: w409 -> [_ w430 _ w444]
      dyn-events: [_ w430 _ w443] -> _
      timeout: w407 -> [_ _ _ _]
      tunnel: [_ TRUE _ _] -> w408
      tunnel: w407 -> [w413 w432 _ _]
      tunnel: [w412 w432 w434 -1 ("Timeout")] -> w406
      tunnel: w403 -> [w414 _ _ _]
      tunnel: [w411 w431 w436 w446] -> w405
      tunnel: w404 -> [w411 w431 _ w446]
      tunnel: [w410 _ w438 w447] -> w402
      event Timeout {
        n171 = event-data() -> ()  [unwired: 1 in, 3 out]
        n172 = disable-structure shown="Enabled" {
          disable-tunnel: w414 -> [w420 _]
          disable-tunnel: w413 -> [w419 w429]
          disable-tunnel: [w418 w429] -> w412
          disable-tunnel: w411 -> [w417 _]
          disable-tunnel: [w416 _] -> w410
          frame Enabled {
            n173 = call "Position reached.vi"("Module ID"=w417) -> ("error out"=w421:errorcluster, "Done?"=w415:bool)  [unwired: 8 in, 1 out]
            n174 = case shown="True" w415 {
              tunnel: w421 -> [w423 w428]
              tunnel: w420 -> [_ w427]
              tunnel: w419 -> [w422 _]
              tunnel: [w422 -1 ("Timeout")] -> w418
              tunnel: w417 -> [_ _]
              tunnel: [w423 w424] -> w416
              frame False {
                # "End-position not reached. Keep asking."
              }
              frame True {
                # "End-position reached. Acquire data."
                n175 = call-poly "Enqueue Message.vi"("error in (no error)"=w428, "Message"="Acquire data", "Message Queue"=w427) -> ("error out"=w424:errorcluster)  [unwired: 7 in, 1 out]
              }
            }
          }
          frame Disabled {
          }
        }
      }
      event User Event {
        n176 = event-data() -> ()  [unwired: 1 in, 1 out]
      }
      event User Event {
        w435 = FALSE  # Echo?
        n177 = event-data() -> ("Timeout"=w434:i32, "Mono Mod ID"=w436:i32, "Wavelength"=w439:dbl)  [unwired: 1 in]
        n178 = disable-structure shown="Disabled" {
          disable-tunnel: [w441 _] -> w437
          disable-tunnel: w436 -> [w440 _]
          frame Disabled {
            n179 = call "Ask position.vi"("Module ID"=w440) -> ("error out"=w441:errorcluster)  [unwired: 8 in, 2 out]
          }
          frame Enabled {
          }
        }
        n180 = call "Move (GOTO).vi"("error in"=w437, "Echo?"=w435, "Position"=w439, "Module ID"=w436) -> ("error out"=w438:errorcluster)  [unwired: 5 in, 2 out]
      }
      event User Event {
        n181 = event-data() -> ("Type"=w442:u32)  [unwired: 1 in]
        n182 = Flush Event Queue(0:w444, 2:w442) -> (8:w443:refnum<event-registration>, 11:w445:errorcluster)  [unwired: 4 in, 1 out]
        n183 = call "Stop movement.vi"("error in"=w445, "Module ID"=w446) -> ("error out"=w447:errorcluster)  [unwired: 9 in]
      }
    }
  }
  n184 = while {
    tunnel: w3 -> [w455]
    shift-right: [w453] -> w27
    shift-left: w24 -> [w454]
    tunnel: [w449] -> w25
    stop <- w451 stop-if-true
    # "Event Handling Loop"
    n185 = event shown="[12] \"Export\": Value Change" {
      selector: w454 -> [_ _ _ _ _ _ _ _ _ _ _ _ _ w512]
      dyn-events: [_ _ _ _ _ _ _ _ _ _ _ _ _ w511] -> w453
      timeout: _ -> [_ _ _ _ _ _ _ _ _ _ _ _ _ _]
      tunnel: [_ _ _ _ _ _ _ TRUE ("Discard?") _ _ _ _ _ _] -> w451
      tunnel: w455 -> [w460 w462 w465 w470 w473 w475 w483 w485 w489 w493 w497 w504 w508 w517]
      tunnel: [w459 _ w466 _ w474 w477 w482 _ w487 w491 w495 w502 w506 w515] -> w452
      tunnel: [w458 w462 w464 w470 w472 w478 w481 w485 w488 w492 w496 w503 w507 w516] -> w450
      event Panel Close? {
        # "Send the 'Confirm Quit' message if the user closes the panel of the VI. Discard the event so the 'Confirm Quit' message has a chance to run."
        n186 = event-data() -> ()  [unwired: 1 in, 1 out]
        n187 = call-poly "Enqueue Message.vi"("Priority Message? (F)"=TRUE, "Message"="Confirm Quit", "Message Queue"=w460) -> ("error out"=w459:errorcluster, "dup Message Queue"=w458:refnum<queue>)  [unwired: 7 in]
        n188 = event-data("Discard?"=TRUE) -> ()  [unwired: 1 in, 1 out]
      }
      event Application Instance Close {
        # "#CodeRecommended - When a project closes, all VIs within that project are aborted and leave memory. However, any code placed in this event frame is guaranteed to run to completion, so add any cleanup code that absolutely must happen here."
        n189 = event-data() -> ()  [unwired: 1 in, 1 out]
      }
      event User Event {
        n190 = event-data() -> ()  [unwired: 1 in, 1 out]
        n191 = call-poly "Enqueue Message.vi"("Message"="Connect Lock-in", "Message Queue"=w465) -> ("error out"=w466:errorcluster, "dup Message Queue"=w464:refnum<queue>)  [unwired: 8 in]
      }
      event User Event {
        w467 = 1000.0  # To mV
        n192 = event-data() -> ("Data"=w469:dbl)  [unwired: 1 in]
        n193 = Multiply(x=w469, y=w467) -> (x*y=→"Current measurement":dbl)
      }
      event User Event {
        n194 = event-data() -> ()  [unwired: 1 in, 1 out]
        n195 = call-poly "Enqueue Message.vi"("Message"="Connect Mono", "Message Queue"=w473) -> ("error out"=w474:errorcluster, "dup Message Queue"=w472:refnum<queue>)  [unwired: 8 in]
      }
      event User Event {
        n196 = event-data() -> ()  [unwired: 1 in, 1 out]
        n197 = call-poly "Enqueue Message.vi"("Message"="Position reached", "Message Queue"=w475) -> ("error out"=w477:errorcluster, "dup Message Queue"=w478:refnum<queue>)  [unwired: 8 in]
      }
      event "Exit": Value Change {
        n198 = event-data() -> ()  [unwired: 1 in, 1 out]
        n199 = call-poly "Enqueue Message.vi"("Priority Message? (F)"=TRUE, "Message"="Exit", "Message Queue"=w483) -> ("error out"=w482:errorcluster, "dup Message Queue"=w481:refnum<queue>)  [unwired: 7 in]
      }
      event User Event {
        # "The Message Handling Loop processed an \"Exit\" message, which fired this event to stop the Event Handling Loop."
        n200 = event-data() -> ()  [unwired: 1 in, 4 out]
      }
      event "Settings": Value Change {
        n201 = event-data() -> ()  [unwired: 1 in, 1 out]
        n202 = call-poly "Enqueue Message.vi"("Message"="Configuration dialog", "Message Queue"=w489) -> ("error out"=w487:errorcluster, "dup Message Queue"=w488:refnum<queue>)  [unwired: 8 in]
      }
      event "Move": Value Change {
        n203 = event-data() -> ()  [unwired: 1 in, 1 out]
        n204 = call-poly "Enqueue Message.vi"("Message"="Move", "Message Queue"=w493) -> ("error out"=w491:errorcluster, "dup Message Queue"=w492:refnum<queue>)  [unwired: 8 in]
      }
      event "Start acquiring": Value Change {
        n205 = event-data() -> ()  [unwired: 1 in, 1 out]
        n206 = call-poly "Enqueue Message.vi"("Message"="Start acquiring", "Message Queue"=w497) -> ("error out"=w495:errorcluster, "dup Message Queue"=w496:refnum<queue>)  [unwired: 8 in]
      }
      event "Continous acquisition": Value Change {
        n207 = event-data() -> ("NewVal"=w501:bool)  [unwired: 1 in]
        n208 = Select(t="Acquire continuously" ("Message"), s=w501, f="Stop continuous acquisition" ("Message")) -> (s? t:f=w498:string)
        n209 = call-poly "Enqueue Message.vi"("Message"=w498, "Message Queue"=w504) -> ("error out"=w502:errorcluster, "dup Message Queue"=w503:refnum<queue>)  [unwired: 8 in]
      }
      event "Export": Value Change {
        n210 = event-data() -> ()  [unwired: 1 in, 1 out]
        n211 = call-poly "Enqueue Message.vi"("Message"="Export to Excel", "Message Queue"=w508) -> ("error out"=w506:errorcluster, "dup Message Queue"=w507:refnum<queue>)  [unwired: 8 in]
      }
      event "Stop acquisition": Value Change {
        n212 = event-data() -> ()  [unwired: 1 in, 1 out]
        n213 = Flush Event Queue(0:w512, 2:lveventtype."User Event" ("event type or object")) -> (8:w511:refnum<event-registration>, 11:w513:errorcluster)  [unwired: 4 in, 1 out]
        n214 = call-poly "Enqueue Message.vi"("Priority Message? (F)"=TRUE, "error in (no error)"=w513, "Message"="Stop acquisition", "Message Queue"=w517) -> ("error out"=w515:errorcluster, "dup Message Queue"=w516:refnum<queue>)  [unwired: 6 in]
      }
    }
    n215 = call "Error Handler - Event Handling Loop.vi"("error in (no error)"=w452, "Message Queue"=w450) -> ("dup error in"=w449:errorcluster)  [unwired: 8 in, 1 out]
  }
  n216 = Unregister For Events(event registration refnum=w27, error in=w25) -> (error out=w28:errorcluster)
  n217 = Merge Errors(w28, w31, w2) -> (w29:errorcluster)
  n218 = call "Destroy User Event - Stop.vi"("error in (no error)"=w29, "User events"=w1) -> ("error out"=w26:errorcluster)  [unwired: 9 in]
  n219 = disable-structure shown="RUN_TIME_ENGINE==True" {
    disable-tunnel: w26 -> [_ _]
    frame condition #0 (active) {
    }
    frame condition #1 {
      # "Call Quit LabVIEW if running as a built application."
      n220 = Quit LabVIEW() -> ()  [unwired: 1 in]
    }
  }
